vi "Tbeam_raw_v2_Main_VI.vi"() -> ()   [LabVIEW 2017]
uses:
  <vilib>/eio/EIONode/EIONode.xnode
  <vilib>/rvi/eio/common/nirviEmuTemplateMethod_errors.vi
  <vilib>/rvi/DataTransferAndStorage/Container/XNode/niFpgaContainer.xnode
  <vilib>/rvi/FIFO/Fifo_Resource/nirvififoEmulationWrite.vi
  <vilib>/rvi/FIFO/Fifo_Resource/nirvififoEmulationRead.vi
  Components/FPGA Functions/FPGA functions.lvlib
  <vilib>/rvi/FXPMathLib/FxpSub/XNode/nifxpmath_Sub.xnode
  <vilib>/rvi/FXPMathLib/FxpMul/XNode/nifxpmath_Multiplier.xnode
  <vilib>/rvi/FXPMathLib/sim/FxpSim.dll
  Components/FPGA Controllers/FPGA Controllers.lvlib
  <vilib>/rvi/FXPMathLib/FxpAdd/XNode/nifxpmath_Add.xnode
panel:
  in  "U_twist dist.":fxp<+/-,25,4>
  in  "U_bend dist.":fxp<+/-,25,4>
  in  "Twist Notch Denominator":fxp<+/-,18,3>[](array[numeric])=[0.0, 0.0]
  in  "Twist Notch Numerator":fxp<+/-,18,3>[](array[numeric])=[0.0, 0.0, 1.0]
  in  "Bend Notch Denominator":fxp<+/-,18,3>[](array[numeric])=[0.0, 0.0]
  in  "Bend Notch Numerator":fxp<+/-,18,3>[](array[numeric])=[0.0, 0.0, 1.0]
  in  "Twist Lead Denominator":fxp<+/-,18,3>[](array[numeric])=[0.0, 0.0]
  in  "Twist Lead Numerator":fxp<+/-,18,3>[](array[numeric])=[0.0, 0.0]
  in  "Bend Lead Denominator":fxp<+/-,18,3>[](array[numeric])=[0.0, 0.0]
  in  "Bend Lead Numerator":fxp<+/-,18,3>[](array[numeric])=[0.0, 0.0]
  in  "Ki*Ts twist":fxp<+,16,0>
  in  "Ki*Ts bend":fxp<+,16,0>
  in  "U_twist [V]":fxp<+/-,26,4>
  in  "U_bend [V]":fxp<+/-,26,4>
  in  "Run controller?":bool
  in  "Kp twist":fxp<+/-,16,10>
  in  "Kp bend":fxp<+/-,16,10>
  in  "Twist reference [V]":fxp<+/-,25,4>
  in  "Bend reference [V]":fxp<+/-,25,4>
  in  "Twist offset [V]":fxp<+/-,26,4>
  in  "Bend offset [V]":fxp<+/-,26,4>
  out "Twist [V]":fxp<+/-,25,4>
  out "Bend [V]":fxp<+/-,25,4>
  in  "AO loop time (Ticks)":u8=222
  in  "Control loop time (Ticks)":u8=10 caption="Control time (us)"
  in  "AI loop time":u8=160 caption="AI loop time (Ticks)"
  out "AO loop time [ticks]":u8
  out "Controller loop [us]":u8
  out "AI proc. time [ticks]":u8
  out "Sample Freq. \ntoo high?":bool
  out "AI Loop time [ticks]":u8
  out "FPGA AI FIFO\nOverflow?":bool
  out "Hall3 [V]":fxp<+,25,3> format="%#.8g"
  out "Hall2 [V]":fxp<+,25,3> format="%#.8g"
  out "AO Coil3 [V]":fxp<+,25,3>
  out "AO Coil2 [V]":fxp<+,25,3>
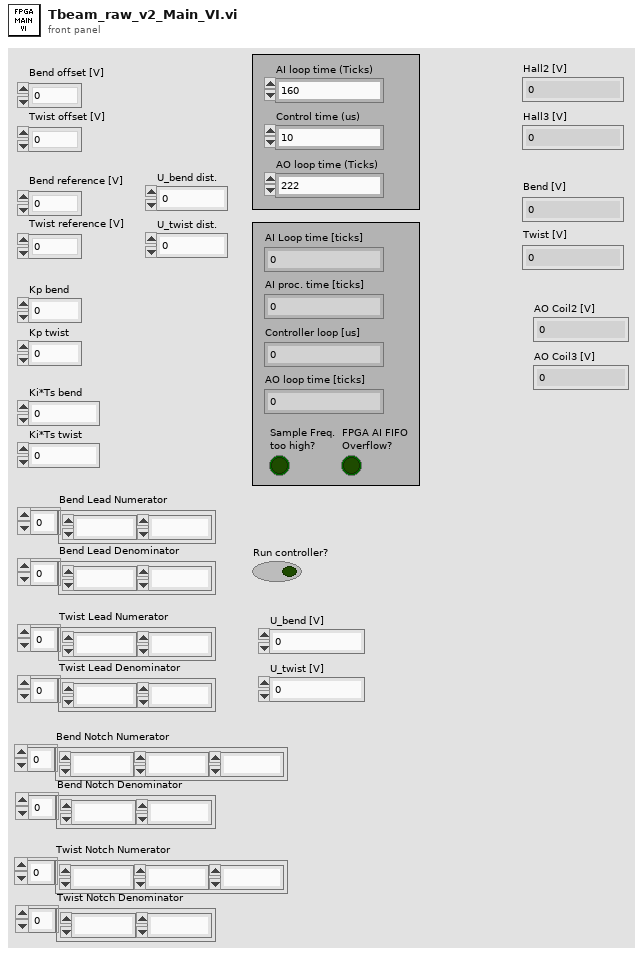
[diagram p1: front panel]
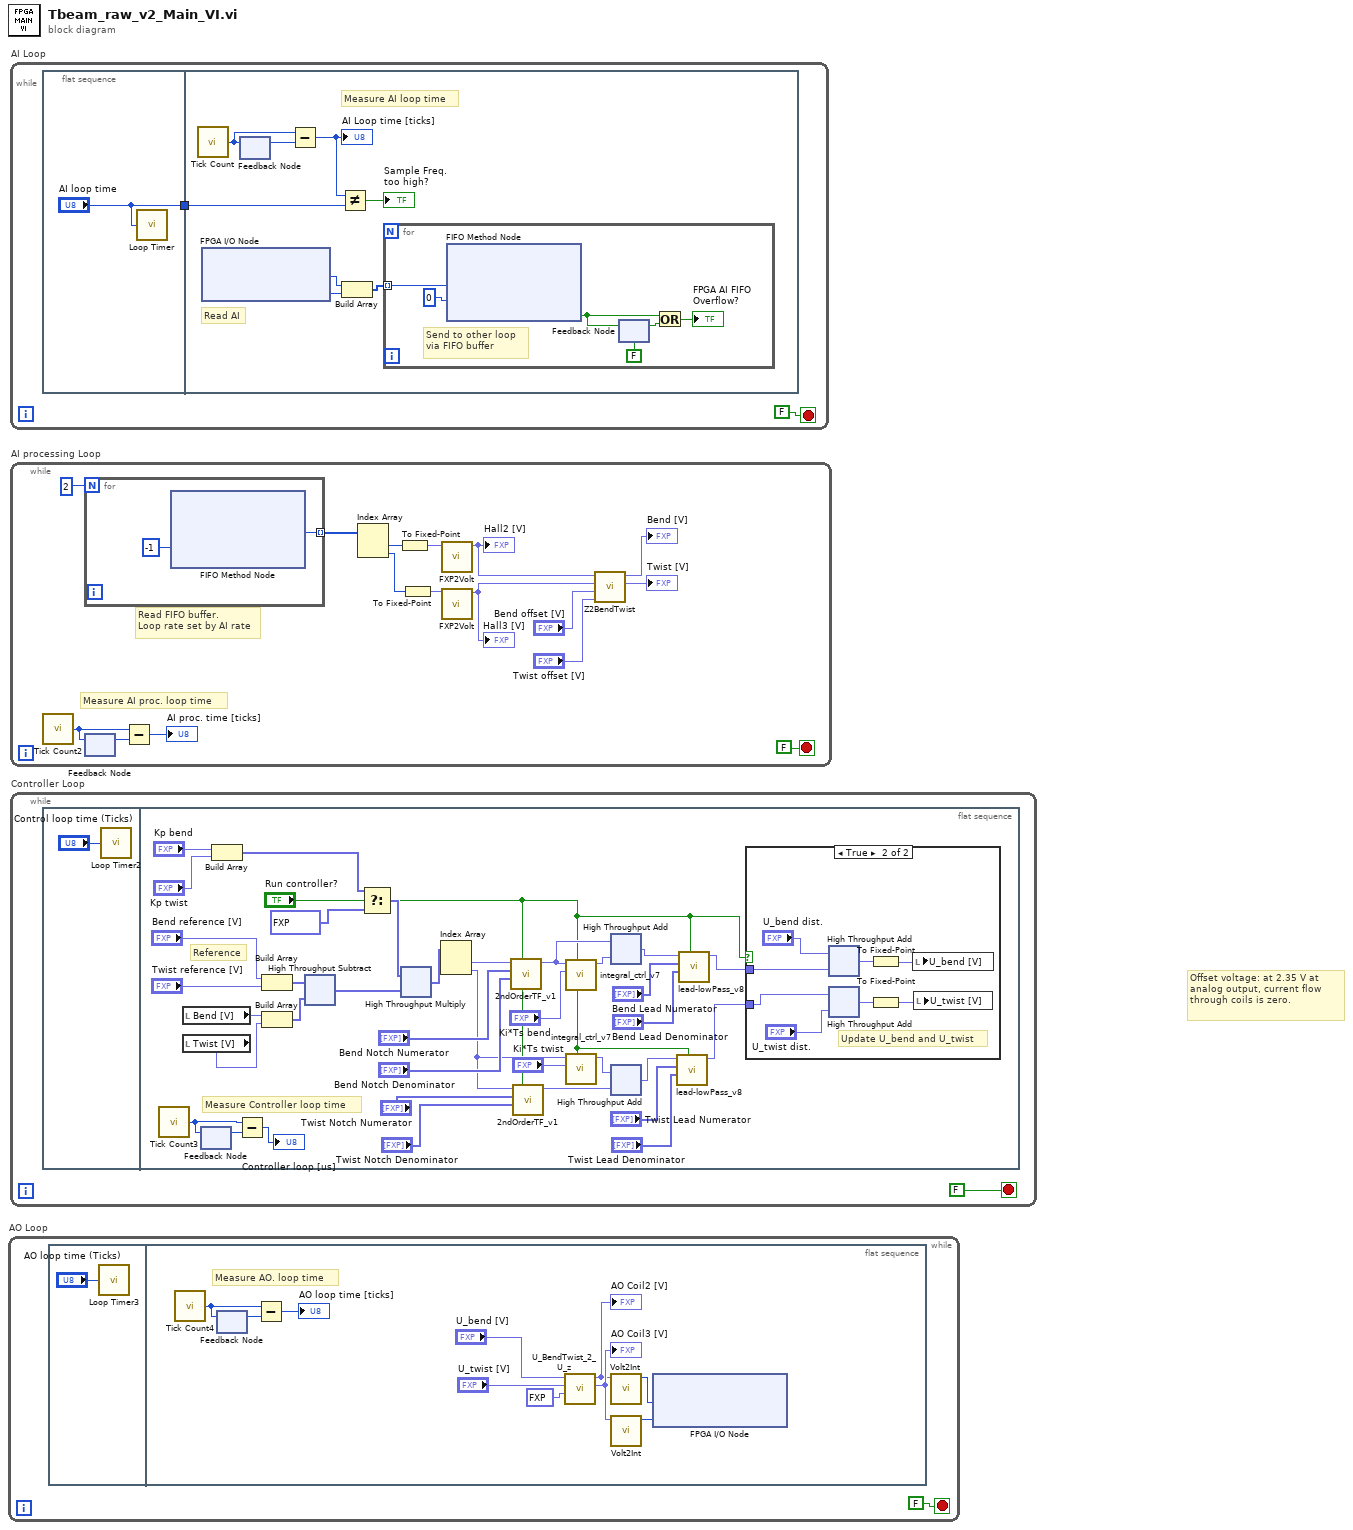
[diagram p0: block diagram]
diagram:
  # "Offset voltage: at 2.35 V at analog output, current flow through coils is zero."
  n1 = while "AO Loop" {
    stop <- FALSE stop-if-true
    n2 = flat-sequence {
      frame #0 {
        n3 = call "Loop Timer3"("Count(Ticks)"="AO loop time (Ticks)") -> ()  [unwired: 1 out]
      }
      frame #1 {
        # "Measure AO. loop time"
        n4 = call "Tick Count4"() -> ("Tick Count(Ticks)"=w12:u8)
        n5 = feedback #1() -> (w11:u8)  [unwired: 1 in]
        n6 = feedback-in #1(w12) -> ()
        n7 = Subtract(x=w12, y=w11) -> (x-y=→"AO loop time [ticks]":u8)
        n8 = call "U_BendTwist_2_U_z.vi"("AO offset [V]"=fxp<+,25,3> 2.3499999046325684, "U_twist [V]"="U_twist [V]", "U_Bend [V]"="U_bend [V]") -> ("AO_coil3 [V]"=w6:fxp<+,25,3>, "AO_coil2 [V]"=w5:fxp<+,25,3>)  [unwired: 7 in]
        "AO Coil2 [V]" <- w5
        "AO Coil3 [V]" <- w6
        n9 = call "Volt2Int.vi"("Input (FXP)"=w5) -> ("Output (Int)"=w8:u16)  [unwired: 10 in]
        n10 = call "Volt2Int.vi"("Input (FXP)"=w6) -> ("Output (Int)"=w9:u16)  [unwired: 10 in]
        n11 = xnode "FPGA I/O Node"("ConnectorB/AO0"=w8, "ConnectorB/AO1"=w9) -> ()  [unwired: 2 in, 2 out]
      }
    }
  }
  n12 = while "AI Loop" {
    stop <- FALSE stop-if-true
    n13 = flat-sequence {
      tunnel: ["AI loop time"] -> w13
      tunnel: w13 -> [w16]
      frame #0 {
        n14 = call "Loop Timer"("Count(Ticks)"="AI loop time") -> ()  [unwired: 1 out]
      }
      frame #1 {
        # "Read AI"
        # "Measure AI loop time"
        n15 = call "Tick Count"() -> ("Tick Count(Ticks)"=w20:u8)
        n16 = xnode "FPGA I/O Node"() -> ("ConnectorB/AI0"=w22:u16, "ConnectorB/AI1"=w23:u16)  [unwired: 2 in, 2 out]
        n17 = feedback #2() -> (w19:u8)  [unwired: 1 in]
        n18 = feedback-in #2(w20) -> ()
        n19 = Subtract(x=w20, y=w19) -> (x-y=w18:u8)
        "AI Loop time [ticks]" <- w18
        n20 = Not Equal?(x=w18, y=w16) -> (x != y?=→"Sample Freq. \ntoo high?":bool)
        n21 = Build Array(w22, w23) -> (w21:u16[])
        n22 = for {
          tunnel: w21 -> [w29] mode=indexing
          # "Send to other loop \nvia FIFO buffer"
          n23 = xnode ("FIFO Method Node")("Element"=w29, "Timeout"=0) -> ("Timed Out?"=w25:bool)  [unwired: 1 in, 1 out]
          n24 = feedback #3(FALSE ("Timed Out?")) -> (w26:bool)
          n25 = feedback-in #3(w25) -> ()
          n26 = Or(x=w25, y=w26) -> (x .or. y?=→"FPGA AI FIFO\nOverflow?":bool)
        }
      }
    }
  }
  n27 = while "AI processing Loop" {
    stop <- FALSE stop-if-true
    # "Measure AI proc. loop time"
    # "Read FIFO buffer.\nLoop rate set by AI rate"
    n28 = call "Tick Count2"() -> ("Tick Count(Ticks)"=w41:u8)
    n29 = for {
      N: 2 -> [_]
      tunnel: [w46] -> w43 mode=indexing
      n30 = xnode ("FIFO Method Node")("Timeout"=-1) -> ("Element"=w46:u16)  [unwired: 1 in, 2 out]
    }
    n31 = feedback #4() -> (w40:u8)  [unwired: 1 in]
    n32 = feedback-in #4(w41) -> ()
    n33 = Subtract(x=w41, y=w40) -> (x-y=→"AI proc. time [ticks]":u8)
    n34 = Index Array(array=w43) -> (element #1=w38:u16, element #2=w30:u16)  [unwired: 2 in]
    n35 = To Fixed-Point(number=w38) -> (fixed-point=w42:fxp<+,22,12>)  [unwired: 1 in]
    n36 = To Fixed-Point(number=w30) -> (fixed-point=w31:fxp<+,22,12>)  [unwired: 1 in]
    n37 = call "FXP2Volt.vi"("Input (Int)"=w42) -> ("Output (FXP)"=w37:fxp<+,25,3>)  [unwired: 10 in]
    "Hall2 [V]" <- w37
    n38 = call "FXP2Volt.vi"("Input (Int)"=w31) -> ("Output (FXP)"=w36:fxp<+,25,3>)  [unwired: 10 in]
    "Hall3 [V]" <- w36
    n39 = call "Z2BendTwist.vi"("Twist offset [V]"="Twist offset [V]", "Bend offset [V]"="Bend offset [V]", "Hall3 [V]"=w36, "Hall2 [V]"=w37) -> ("Twist [V]"=→"Twist [V]":fxp<+/-,25,4>, "Bend [V]"=→"Bend [V]":fxp<+/-,25,4>)  [unwired: 6 in]
  }
  n40 = while "Controller Loop" {
    stop <- FALSE stop-if-true
    n41 = flat-sequence {
      frame #0 {
        n42 = call "Loop Timer2"("Count(uSec)"="Control loop time (Ticks)") -> ()  [unwired: 1 out]
      }
      frame #1 {
        # "Measure Controller loop time"
        # "Reference"
        n43 = call "Tick Count3"() -> ("Tick Count(uSec)"=w86:u8)
        n44 = local read "Bend [V]"() -> (w81:fxp<+/-,25,4>)
        n45 = local read "Twist [V]"() -> (w80:fxp<+/-,25,4>)
        n46 = feedback #5() -> (w85:u8)  [unwired: 1 in]
        n47 = feedback-in #5(w86) -> ()
        n48 = Build Array("Kp bend", "Kp twist") -> (w74:fxp<+/-,16,10>[])
        n49 = Subtract(x=w86, y=w85) -> (x-y=→"Controller loop [us]":u8)
        n50 = Build Array("Bend reference [V]", "Twist reference [V]") -> (w79:fxp<+/-,25,4>[])
        n51 = Build Array(w81, w80) -> (w78:fxp<+/-,25,4>[])
        n52 = xnode "High Throughput Subtract"("x"=w79, "y"=w78) -> ("x-y"=w77:fxp<+/-,25,4>[])
        n53 = Select(t=w74, s="Run controller?", f=fxp<+/-,16,10>[] [0.0, 0.0]) -> (s? t:f=w75:fxp<+/-,16,10>[])
        n54 = xnode ("High Throughput Multiply")("x"=w75, "y"=w77) -> ("x*y"=w76:fxp<+/-,25,4>[])
        n55 = Index Array(array=w76) -> (element #1=w58:fxp<+/-,25,4>, element #2=w54:fxp<+/-,25,4>)  [unwired: 2 in]
        n56 = call "2ndOrderTF_v1.vi"("Enable?"="Run controller?", "Denominator"="Bend Notch Denominator", "Numerator"="Bend Notch Numerator", "Input"=w58) -> ("Output"=w57:fxp<+/-,25,4>)  [unwired: 7 in]
        n57 = call "2ndOrderTF_v1.vi"("Enable?"="Run controller?", "Denominator"="Twist Notch Denominator", "Numerator"="Twist Notch Numerator", "Input"=w54) -> ("Output"=w53:fxp<+/-,25,4>)  [unwired: 7 in]
        n58 = call "integral_ctrl_v7.vi"("Enable?"="Run controller?", "Ki*Ts"="Ki*Ts bend", "Input"=w57) -> ("Output"=w67:fxp<+/-,25,4>)  [unwired: 8 in]
        n59 = call "integral_ctrl_v7.vi"("Enable?"="Run controller?", "Ki*Ts"="Ki*Ts twist", "Input"=w54) -> ("Output"=w68:fxp<+/-,25,4>)  [unwired: 8 in]
        n60 = xnode ("High Throughput Add")("x"=w57, "y"=w67) -> ("x+y"=w66:fxp<+/-,25,4>)
        n61 = xnode ("High Throughput Add")("x"=w68, "y"=w53) -> ("x+y"=w65:fxp<+/-,25,4>)
        n62 = call "lead-lowPass_v8.vi"("Enable?"="Run controller?", "Denominator"="Twist Lead Denominator", "Numerator"="Twist Lead Numerator", "Input"=w65) -> ("Output"=w63:fxp<+/-,25,4>)  [unwired: 7 in]
        n63 = call "lead-lowPass_v8.vi"("Enable?"="Run controller?", "Denominator"="Bend Lead Denominator", "Numerator"="Bend Lead Numerator", "Input"=w66) -> ("Output"=w64:fxp<+/-,25,4>)  [unwired: 7 in]
        n64 = case shown="True" "Run controller?" {
          tunnel: w64 -> [_ w92]
          tunnel: w63 -> [_ w87]
          frame False {
          }
          frame True {
            # "Update U_bend and U_twist"
            n65 = xnode "High Throughput Add"("x"="U_bend dist.", "y"=w92) -> ("x+y"=w91:fxp<+/-,26,5>)
            n66 = xnode "High Throughput Add"("x"=w87, "y"="U_twist dist.") -> ("x+y"=w90:fxp<+/-,26,5>)
            n67 = To Fixed-Point(number=w91) -> (fixed-point=w94:fxp<+/-,26,4>)  [unwired: 1 in]
            n68 = To Fixed-Point(number=w90) -> (fixed-point=w93:fxp<+/-,26,4>)  [unwired: 1 in]
            n69 = local write "U_bend [V]"(w94) -> ()
            n70 = local write "U_twist [V]"(w93) -> ()
          }
        }
      }
    }
  }
